vi "Remove Outliers (multiple).vi"(8 "error in (no error)":errorcluster, 9 "Y Lower":dbl, 10 "Y Upper":dbl, 11 "XY-data":cluster{"X-array":dbl[], "Y-array":dbl[]}[](array[cluster])) -> (0 "error out":errorcluster, 3 "XY-data out":cluster{"X-array":dbl[], "Y-array":dbl[]}[](array[cluster]) {"Y-array" format="%.2p"; "X-array" format="%.2p"})   [LabVIEW 2019, in "xy_utilities.lvlib"]
doc: "Remove outliers from the y array of <b>XY-data</b> between <b>Y Upper</b> and <b>Y Lower</b> limits.\n\nWire data to the data input to determine the polymorphic instance to use or manually select the instance."
uses:
  xy_utilities.lvlib
  <vilib>/Analysis/6fits.llb/Remove Outliers.vi
  <vilib>/Analysis/6fits.llb/Remove Outliers (Range).vi
  <vilib>/Utility/error.llb/Error Cluster From Error Code.vi
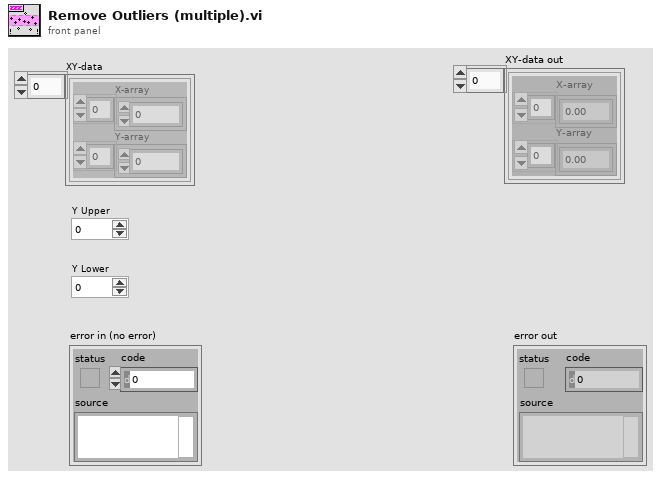
[diagram p1: front panel]
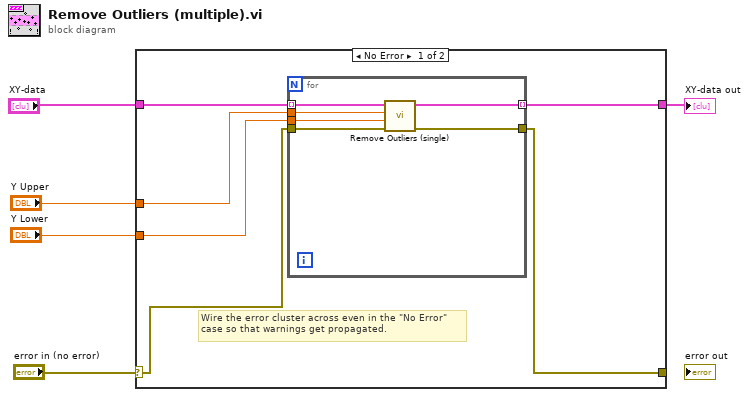
[diagram p0: block diagram]
diagram:
  n1 = case shown="No Error" "error in (no error)" {
    selector: "error in (no error)" -> [w10 w18]
    tunnel: [w11 w18] -> _
    tunnel: "Y Lower" -> [w9 _]
    tunnel: "Y Upper" -> [w8 _]
    tunnel: "XY-data" -> [w7 w19]
    tunnel: [w6 w19] -> w1
    frame No Error {
      # "Wire the error cluster across even in the \"No Error\"\ncase so that warnings get propagated."
      n2 = for {
        tunnel: w9 -> [w15]
        tunnel: w8 -> [w16]
        tunnel: w7 -> [w17] mode=indexing
        tunnel: [w12] -> w6 mode=indexing
        tunnel: w10 -> [w14]
        tunnel: [w13] -> w11
        n3 = call "Remove Outliers (single).vi"("error in (no error)"=w14, "Y Lower"=w15, "Y Upper"=w16, "XY-data"=w17) -> ("error out"=w13:errorcluster, "XY-data out"=w12:cluster{"X-array":dbl[], "Y-array":dbl[]})  [unwired: 6 in]
      }
    }
    frame Error {
    }
  }
  "XY-data out" <- w1
